vi "instr.ATF20D+.vi"(5 "Unit":T1(ring), 6 "Para":dbl, 7 "timeout (10sec)":u32=2000 caption="超时（10秒）", 8 "error in (no error)":errorcluster caption="错误输入（无错误）", 9 "CMD":enum16{"FREQ", "VPP", "VRMS", "SWITCH"}(ring), 10 "Channel":enum16{"CHA", "CHB", "Connect", "DisConnect"}(ring), 11 "VISA resource name":refnum<visa-resource-name> caption="VISA资源名称") -> (0 "error out":errorcluster caption="错误输出", 1 "Reply Str":string, 2 "CMD Str":string, 3 "OK?":bool, 4 "VISA.Output":refnum<visa-resource-name> caption="VISA.output")   [LabVIEW 2012, in "Lib_UEL.ATE.lvlib" / "Lib_Instrument.lvlib"]
uses:
  Lib_Instrument.lvlib
  <vilib>/Instr/_visa.llb/VISA Configure Serial Port (Instr).vi
panel:
  in  "Address":u8=88 format="%02.0f"
  # "- 设置幅度输出时，需要加入带负载的修正值。\n- 不要使用USBTORS232来操作信号源。"
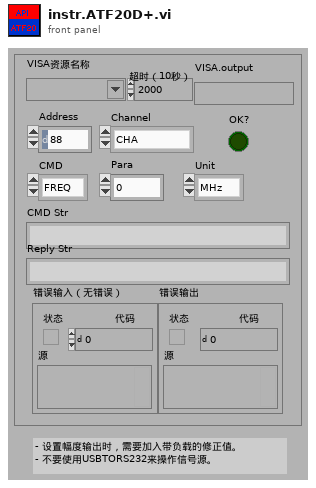
[diagram p1: front panel]
types:
  T1 = enum16{"MHz", "kHz", "Hz", "Vpp", "mVpp", "Vrms", "mVrms", "No."}
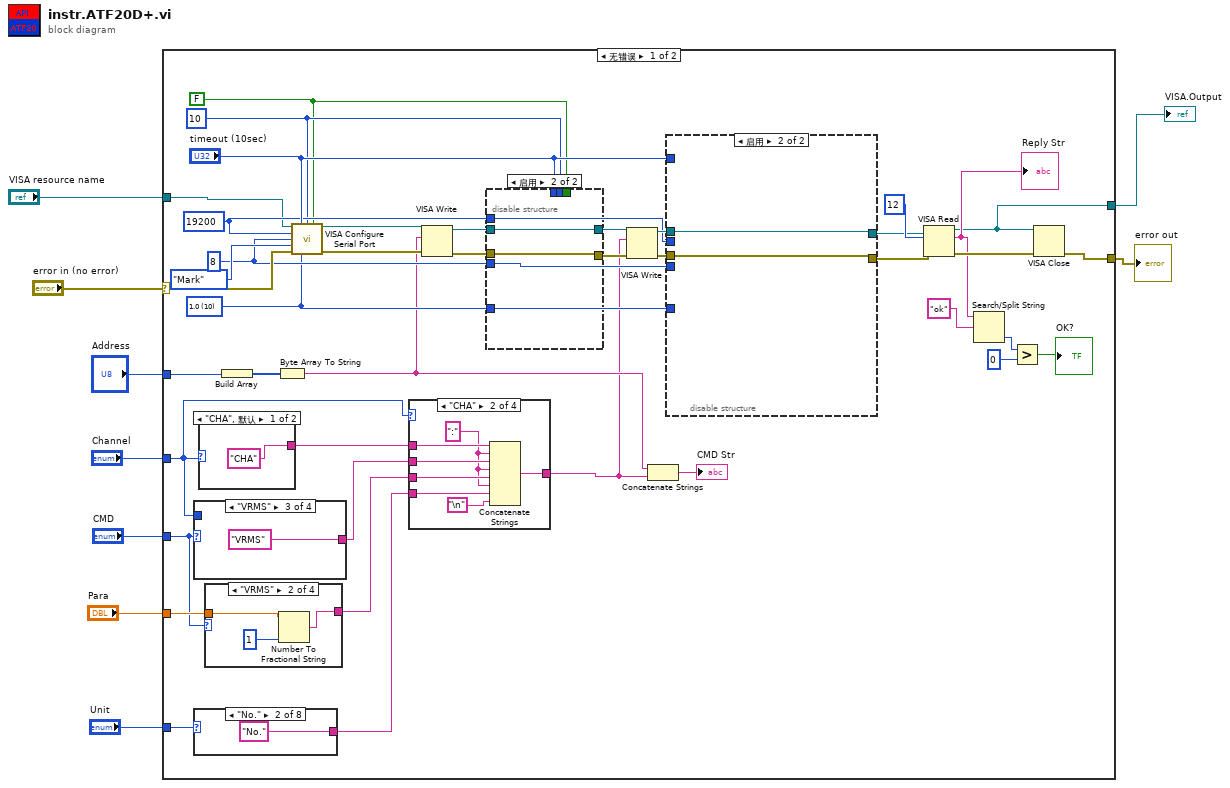
[diagram p0: block diagram]
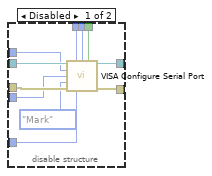
[diagram p2: hidden frame]
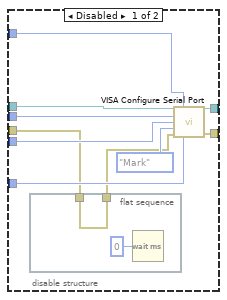
[diagram p3: hidden frame]
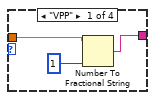
[diagram p4: hidden frame]
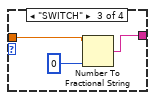
[diagram p5: hidden frame]
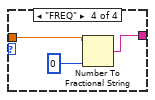
[diagram p6: hidden frame]
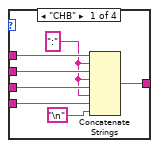
[diagram p7: hidden frame]
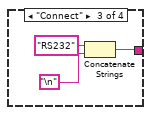
[diagram p8: hidden frame]
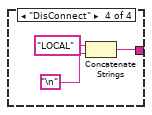
[diagram p9: hidden frame]
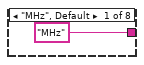
[diagram p10: hidden frame]
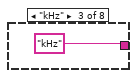
[diagram p11: hidden frame]
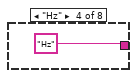
[diagram p12: hidden frame]
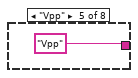
[diagram p13: hidden frame]
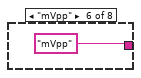
[diagram p14: hidden frame]
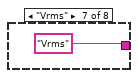
[diagram p15: hidden frame]
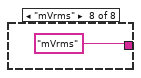
[diagram p16: hidden frame]
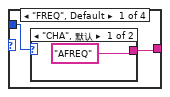
[diagram p17: hidden frame]
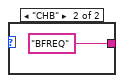
[diagram p18: hidden frame]
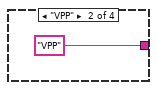
[diagram p19: hidden frame]
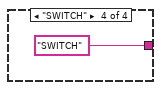
[diagram p20: hidden frame]
diagram:
  n1 = case shown="无错误" "error in (no error)" {
    selector: "error in (no error)" -> [w50 w128]
    tunnel: [w48 w128] -> w8
    tunnel: "Address" -> [w47 _]
    tunnel: "Channel" -> [w19 _]
    tunnel: "CMD" -> [w12 _]
    tunnel: "Para" -> [w13 _]
    tunnel: "Unit" -> [w23 _]
    tunnel: [w11 w127] -> w2
    tunnel: "VISA resource name" -> [w10 w127]
    frame No Error {
      w30 = u8 10 ("termination char\n(0xA = '\\n' = LF)")
      w33 = u16 10 items=["1.0"=10, "1.5"=15, "2.0"=20] ("stop bits (10: 1 bit)")
      w34 = u16 8 ("data bits (8)")
      w29 = FALSE ("Enable Termination\nChar (T)")
      w35 = u32 19200 ("baud rate (9600)")
      n2 = case shown="\"VRMS\"" w12 {
        tunnel: [w118 "VPP" "VRMS" "SWITCH"] -> w25
        tunnel: w19 -> [w119 _ _ _]
        frame "FREQ", Default {
          n3 = case shown="\"CHA\", 默认" w119 {
            tunnel: ["AFREQ" "BFREQ"] -> w118
            frame "CHA", Default {
            }
            frame "CHB" {
            }
          }
        }
        frame "VPP" {
        }
        frame "VRMS" {
        }
        frame "SWITCH" {
        }
      }
      n4 = case shown="\"No.\"" w23 {
        tunnel: ["MHz" "No." "kHz" "Hz" "Vpp" "mVpp" "Vrms" "mVrms"] -> w22
        frame "MHz", Default {
        }
        frame "No." {
        }
        frame "kHz" {
        }
        frame "Hz" {
        }
        frame "Vpp" {
        }
        frame "mVpp" {
        }
        frame "Vrms" {
        }
        frame "mVrms" {
        }
      }
      n5 = case shown="\"CHA\", 默认" w19 {
        tunnel: ["CHA" "CHB"] -> w26
        frame "CHA", Default {
        }
        frame "CHB" {
        }
      }
      n6 = case shown="\"VRMS\"" w12 {
        tunnel: [w80 w83 w86 w89] -> w24
        tunnel: w13 -> [w79 w82 w85 w88]
        frame "VPP" {
          n7 = Number To Fractional String(number=w79, precision (6)=i16 1 ("精度(6)")) -> (F-format string=w80:string)  [unwired: 2 in]
        }
        frame "VRMS" {
          n8 = Number To Fractional String(number=w82, precision (6)=i16 1 ("精度(6)")) -> (F-format string=w83:string)  [unwired: 2 in]
        }
        frame "SWITCH" {
          n9 = Number To Fractional String(number=w85, precision (6)=i16 0 ("精度(6)")) -> (F-format string=w86:string)  [unwired: 2 in]
        }
        frame "FREQ" {
          n10 = Number To Fractional String(number=w88, precision (6)=i16 0 ("精度(6)")) -> (F-format string=w89:string)  [unwired: 2 in]
        }
      }
      n11 = Build Array(w47) -> (w46:u8[])
      n12 = Byte Array To String(unsigned byte array=w46) -> (string=w28:string)
      n13 = call-poly "VISA Configure Serial Port"("VISA resource name"=w10, "timeout (10sec)"="timeout (10sec)", "termination char\n(0xA = '\\n' = LF)"=w30, "Enable Termination\nChar (T)"=w29, "baud rate (9600)"=w35, "data bits (8)"=w34, "parity (0:none)"=enum16{"None", "Odd", "Even", "Mark", "Space"}."Mark", "error in (no error)"=w50, "stop bits (10: 1 bit)"=w33) -> ("VISA resource name out"=w43:refnum<visa-resource-name>, "error out"=w44:errorcluster)  [unwired: 5 in]
      n14 = case shown="\"CHA\"" w19 {
        tunnel: w26 -> [w96 w103 _ _]
        tunnel: w25 -> [w95 w102 _ _]
        tunnel: w24 -> [w94 w101 _ _]
        tunnel: w22 -> [w92 w99 _ _]
        tunnel: [w91 w98 w106 w109] -> w21
        frame "CHB" {
          w93 = ":"
          n15 = Concatenate Strings(w96, w93, w95, w93, w94, w93, w92, "\n") -> (w91:string)
        }
        frame "CHA" {
          w100 = ":"
          n16 = Concatenate Strings(w103, w100, w102, w100, w101, w100, w99, "\n") -> (w98:string)
        }
        frame "Connect" {
          n17 = Concatenate Strings("RS232" ("字符串"), "\n") -> (w106:string)
        }
        frame "DisConnect" {
          n18 = Concatenate Strings("LOCAL" ("字符串"), "\n") -> (w109:string)
        }
      }
      n19 = VISA Write(VISA resource name=w43, write buffer=w28, error in (no error)=w44) -> (VISA resource name out=w38:refnum<visa-resource-name>, error out=w42:errorcluster)  [unwired: 1 out]
      n20 = disable-structure shown="启用" {
        disable-tunnel: w42 -> [w61 w62]
        disable-tunnel: [w60 w63] -> w41
        disable-tunnel: [w59 w62] -> w40
        disable-tunnel: w38 -> [w57 w63]
        disable-tunnel: "timeout (10sec)" -> [w56 _]
        disable-tunnel: w35 -> [w55 _]
        disable-tunnel: w34 -> [w54 _]
        disable-tunnel: w33 -> [w53 _]
        disable-tunnel: w30 -> [w52 _]
        disable-tunnel: w29 -> [w51 _]
        frame Disabled {
          n21 = call-poly "VISA Configure Serial Port"("VISA resource name"=w57, "timeout (10sec)"=w56, "termination char\n(0xA = '\\n' = LF)"=w52, "Enable Termination\nChar (T)"=w51, "baud rate (9600)"=w55, "data bits (8)"=w54, "parity (0:none)"=enum16{"None", "Odd", "Even", "Mark", "Space"}."Mark", "error in (no error)"=w61, "stop bits (10: 1 bit)"=w53) -> ("VISA resource name out"=w60:refnum<visa-resource-name>, "error out"=w59:errorcluster)  [unwired: 5 in]
        }
        frame Enabled {
        }
      }
      n22 = VISA Write(VISA resource name=w41, write buffer=w21, error in (no error)=w40) -> (VISA resource name out=w37:refnum<visa-resource-name>, error out=w20:errorcluster)  [unwired: 1 out]
      n23 = Concatenate Strings(w28, w21) -> (→"CMD Str":string)
      n24 = disable-structure shown="启用" {
        disable-tunnel: w37 -> [w73 w77]
        disable-tunnel: "timeout (10sec)" -> [w72 _]
        disable-tunnel: w35 -> [w71 _]
        disable-tunnel: w34 -> [w70 _]
        disable-tunnel: w33 -> [w69 _]
        disable-tunnel: [w68 w77] -> w32
        disable-tunnel: [w67 w76] -> w31
        disable-tunnel: w20 -> [w64 w76]
        frame Disabled {
          n25 = flat-sequence {
            tunnel: [w75] -> w65
            tunnel: w64 -> [w75]
            frame #0 {
              n26 = Wait (ms)(milliseconds to wait=u32 0 ("等待时间（毫秒）")) -> ()  [unwired: 1 out]
            }
          }
          n27 = call-poly "VISA Configure Serial Port"("VISA resource name"=w73, "timeout (10sec)"=w72, "baud rate (9600)"=w71, "data bits (8)"=w70, "parity (0:none)"=enum16{"None", "Odd", "Even", "Mark", "Space"}."Mark", "error in (no error)"=w65, "stop bits (10: 1 bit)"=w69) -> ("VISA resource name out"=w68:refnum<visa-resource-name>, "error out"=w67:errorcluster)  [unwired: 7 in]
        }
        frame Enabled {
        }
      }
      n28 = VISA Read(VISA resource name=w32, byte count=u32 12 ("字节总数"), error in (no error)=w31) -> (VISA resource name out=w11:refnum<visa-resource-name>, read buffer=w18:string, error out=w49:errorcluster)  [unwired: 1 out]
      "Reply Str" <- w18
      n29 = Search/Split String(string=w18, search string/char (-)="ok" ("搜索字符串")) -> (offset of match=w16:i32)  [unwired: 1 in, 2 out]
      n30 = Greater?(x=w16, y=0) -> (0:→"OK?":bool)
      n31 = VISA Close(VISA resource name=w11, error in (no error)=w49) -> (error out=w48:errorcluster)
    }
    frame Error {
    }
  }
  "error out" <- w8
  "VISA.Output" <- w2
